vi "Begin.vi"(11 "Image Size":T1=enum."320x240") -> (0 "error out":errorcluster)   [LabVIEW 2011]
doc: "Called before other user functions, this VI is expected to open initial I/O refnums, load in file data, and do all program initialization. Notice that the <B>error out</B> terminal is simply used for data flow. Wiring it to other structures or subVIs ensures that this VI runs first."
uses:
  <vilib>/Rock Robotics/WPI/Camera/WPI_CameraImageSize.ctl
  <vilib>/Rock Robotics/SystemInterfaces/DIO/FPGA_DIOPWMChannel.ctl
  <vilib>/Rock Robotics/WPI/Joystick/WPI_JoystickDeviceEnum.ctl
  <vilib>/Rock Robotics/SystemInterfaces/DIO/FPGA_DIOChannel.ctl
  <vilib>/Rock Robotics/SystemInterfaces/DIO/FPGA_DIORelayChannel.ctl
  <vilib>/Rock Robotics/WPI/Solenoid/WPI_SolenoidChannel.ctl
  <vilib>/Rock Robotics/SystemInterfaces/Typedef/FPGA_TypedefAnalogModuleForGyro.ctl
  <vilib>/Rock Robotics/SystemInterfaces/AI/FPGA_AIGyroChannel.ctl
  <vilib>/Rock Robotics/SystemInterfaces/Typedef/FPGA_TypedefSolenoidModule.ctl
  <vilib>/Rock Robotics/SystemInterfaces/Typedef/FPGA_TypedefDigitalModule.ctl
  <vilib>/Rock Robotics/WPI/CAN/Jaguar/SubVIs/WPI_CANJaguar_ControlMode.ctl
  <vilib>/Rock Robotics/SystemInterfaces/Typedef/FPGA_TypedefAnalogModule.ctl
  <vilib>/Rock Robotics/SystemInterfaces/AI/FPGA_AIChannel.ctl
  <vilib>/Rock Robotics/WPI/Camera/WPI_CameraWhite Balance Values.ctl
  <vilib>/Rock Robotics/WPI/Camera/WPI_CameraExposure Values.ctl
  <vilib>/Rock Robotics/WPI/Encoder/WPI_EncoderType.ctl
  <vilib>/Rock Robotics/WPI/Camera/WPI_CameraFrameRate.ctl
  <vilib>/Rock Robotics/WPI/CAN/Jaguar/SubVIs/WPI_CANJaguar_BrakeCoastMode.ctl
  <vilib>/Rock Robotics/WPI/CAN/Jaguar/SubVIs/WPI_CANJaguar_LimitMode.ctl
  <vilib>/Rock Robotics/WPI/CAN/Jaguar/SubVIs/WPI_CANJaguar_PositionReference.ctl
  <vilib>/Rock Robotics/WPI/CAN/Jaguar/SubVIs/WPI_CANJaguar_StatusSelect.ctl
  <vilib>/Rock Robotics/WPI/CAN/Jaguar/SubVIs/WPI_CANJaguar_StatusChannelSelect.ctl
  <vilib>/Rock Robotics/WPI/RobotDrive/WPI_RobotDriveOpen4MotorWithVictor.vi
  <vilib>/Rock Robotics/WPI/Solenoid/WPI_SolenoidOpenSingle.vi
  <vilib>/Rock Robotics/WPI/MotorControl/WPI_MotorControlOpen Victor.vi
  <vilib>/Rock Robotics/WPI/RobotDrive/WPI_RobotDriveOpen2MotorWithExistingMotors.vi
  <vilib>/Rock Robotics/WPI/Counter/WPI_CounterDigitalInputToDigitalSource.vi
  Robot Global Data.vi
  <vilib>/Rock Robotics/WPI/MotorControl/WPI_MotorControlOpenCANJaguar.vi
  <vilib>/Rock Robotics/WPI/Compressor/WPI_CompressorGetSetRefNum.vi
panel:
  out "error out 2":errorcluster
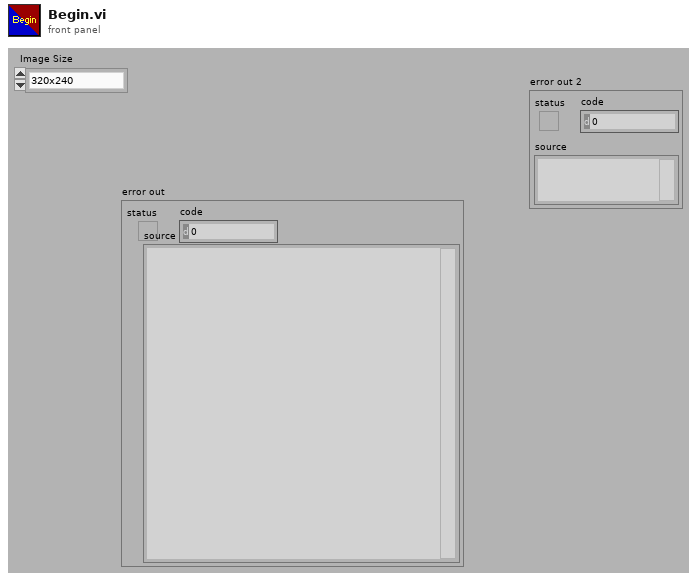
[diagram p1: front panel]
types:
  T1 = typedef "WPI_CameraImageSize.ctl" = enum16{"640x480", "320x240", "160x120"}
  T2 = typedef "WPI_CameraFrameRate.ctl" = u32
  T3 = typedef "FPGA_DIOChannel.ctl" = enum8{"DIO 1", "DIO 2", "DIO 3", "DIO 4", "DIO 5", "DIO 6", "DIO 7", "DIO 8", "DIO 9", "DIO 10", "DIO 11", "DIO 12", "DIO 13", "DIO 14", "Invalid"}
  T4 = typedef "FPGA_TypedefDigitalModule.ctl" = enum16{"Digital Module 1", "Digital Module 2"}
  T5 = typedef "WPI_EncoderType.ctl" = enum16{"1x", "2x", "4x"}
  T6 = typedef "WPI_CameraExposure Values.ctl" = enum16{"Auto", "Flicker-free 50 Hz", "Flicker-free 60 Hz", "Hold current"}
  T7 = typedef "WPI_CameraWhite Balance Values.ctl" = enum16{"Auto", "Fixed indoor", "Fixed outdoor 1", "Fixed outdoor 2", "Fixed fluorescent 1", "Fixed fluorescent 2", "Hold current"}
  T8 = typedef "WPI_SolenoidChannel.ctl" = enum8{"Solenoid 1", "Solenoid 2", "Solenoid 3", "Solenoid 4", "Solenoid 5", "Solenoid 6", "Solenoid 7", "Solenoid 8", "Invalid"}
  T9 = typedef "FPGA_TypedefSolenoidModule.ctl" = enum16{"Solenoid Module 1", "Solenoid Module 2"}
  T10 = typedef "FPGA_AIChannel.ctl" = enum8{"AI 1", "AI 2", "AI 3", "AI 4", "AI 5", "AI 6", "AI 7", "AI 8", "Invalid"}
  T11 = typedef "FPGA_TypedefAnalogModule.ctl" = enum16{"Analog Module 1", "Analog Module 2"}
  T12 = typedef "WPI_CANJaguar_ControlMode.ctl" = enum8{"Percent VBus", "Current", "Speed", "Position", "Voltage"}
  T13 = typedef "FPGA_DIOPWMChannel.ctl" = enum8{"PWM 1", "PWM 2", "PWM 3", "PWM 4", "PWM 5", "PWM 6", "PWM 7", "PWM 8", "PWM 9", "PWM 10", "Invalid"}
  T14 = typedef "FPGA_AIGyroChannel.ctl" = enum8{"AI 1", "AI 2", "Invalid"}
  T15 = typedef "FPGA_TypedefAnalogModuleForGyro.ctl" = enum16{"Analog Module 1"}
  T16 = typedef "WPI_JoystickDeviceEnum.ctl" = enum16{"USB 1", "USB 2", "USB 3", "USB 4", "Kinect 1", "Kinect 2"}
  T17 = typedef "FPGA_DIORelayChannel.ctl" = enum8{"Relay 1", "Relay 2", "Relay 3", "Relay 4", "Relay 5", "Relay 6", "Relay 7", "Relay 8", "Invalid"}
  T18 = typedef "WPI_AnalogChannelDevRef.ctl" = cluster{"DevStatus":errorcluster, "Analog Module":T11, "Analog Channel":T10}
  T19 = typedef "WPI_DigitalInputDevRef.ctl" = cluster{"DevStatus":errorcluster, "DIO Channel":T3, "Digital Module":T4}
  T20 = typedef "WPI_GyroDevRef.ctl" = cluster{"DevStatus":errorcluster, "Analog Module":T11, "Analog Channel":T10, "Offset":dbl, "Gain (VoltsPerDegree/Second)":dbl}
  T21 = typedef "FPGA_CounterEncoderSourceConvertionLVSourceType.ctl" = cluster{"DevStatus":errorcluster, "AnalogTriggerMode?":bool, "DigitalMode":cluster{"Digital Module":T4, "DIO Channel":T22}, "AnalogTriggerMode":cluster{"AnalogTriggerIndex":T23, "OutputType":T24}}
  T22 = typedef "FPGA_DIODigitalSourceChannel.ctl" = enum8{"DIO 1", "DIO 2", "DIO 3", "DIO 4", "DIO 5", "DIO 6", "DIO 7", "DIO 8", "DIO 9", "DIO 10", "DIO 11", "DIO 12", "DIO 13", "DIO 14", "Disabled"}
  T23 = typedef "FPGA_AnalogTriggerIndex.ctl" = enum8{"Trig 0", "Trig 1", "Trig 2", "Trig 3", "Trig 4", "Trig 5", "Trig 6", "Trig 7", "Invalid"}
  T24 = typedef "FPGA_AnalogTriggerOutType.ctl" = enum16{"InWindow", "TriggerState", "Rising", "Falling"}
  T25 = typedef "WPI_EncoderDevRef.ctl" = cluster{"DevStatus":errorcluster, "EncoderIndex":T26, "CounterIndex":T27, "DistancePerCount":dbl, "Decoding Type":T5}
  T26 = typedef "FPGA_EncoderIdx.ctl" = enum8{"Enc 0", "Enc 1", "Enc 2", "Enc 3", "Invalid"}
  T27 = typedef "FPGA_CounterCtrSystemIndex.ctl" = enum8{"Ctr 0", "Ctr 1", "Ctr 2", "Ctr 3", "Ctr 4", "Ctr 5", "Ctr 6", "Ctr 7", "Invalid"}
  T28 = typedef "WPI_CameraDevRef.ctl" = cluster{"Camera Address":string, "CameraStatus":errorcluster, "Acquire Image Notifier":refnum<notifier>}
  T29 = typedef "WPI_CompressorDevRef.ctl" = cluster{"DevStatus":errorcluster, "DigitalInputDevRef":T19, "RelayDevRef":T30}
  T30 = typedef "WPI_RelayDevRef.ctl" = cluster{"DevStatus":errorcluster, "Relay Channel":T17, "Digital Module":T4, "Relay Direction":T31}
  T31 = typedef "WPI_RelayDirection.ctl" = enum16{"Both directions", "Forward only", "Reverse only"}
  T32 = typedef "WPI_MotorControlDeviceRef.ctl" = cluster{"DeviceStatus":errorcluster, "Type":enum16{"PWM", "CAN"}, "PWM":cluster{"Digital Module":T4, "PWM Channel":T13, "DeadBand":T33}, "CAN":cluster{"Device Number":u8, "Control Mode":T12, "Semaphore":T34, "Max Vout":dbl}, "Invert":bool, "TransformRef":T35, "InvTransformRef":T35}
  T33 = typedef "WPI_PWMDeadband.ctl" = cluster{"Name":string, "maxPositivePwm":i32, "minPositivePwm":i32, "centerPwm":i32, "maxNegativePwm":i32, "minNegativePwm":i32, "angularRange":u16}
  T34 = typedef "Semaphore RefNum" = refnum<k1>
  T35 = typedef "WPI_PWMTransform_ConPane.ctl" = refnum<vi>
  T36 = typedef "WPI_DigitalOutputDevRef.ctl" = cluster{"Digital Module":T4, "DIO Channel":T3, "DevStatus":errorcluster}
  T37 = typedef "WPI_SolenoidDevRef.ctl" = cluster{"DevStatus":errorcluster, "Solenoid Module":T9, "Forward Solenoid Channel":T8, "Reverse Solenoid Channel":T8}
  T38 = typedef "WPI_JoystickDevRef.ctl" = cluster{"Device":T16}
  T39 = typedef "WPI_RobotDriveDevRef.ctl" = cluster{"DevStatus":errorcluster, "Motors[]":T32[], "Square Inputs":bool, "Max Output":dbl, "Isochronous":bool}
  T40 = typedef "WPI_CANJaguar_BrakeCoastMode.ctl" = enum8{"Jumper", "Brake", "Coast"}
  T41 = typedef "WPI_CANJaguar_LimitMode.ctl" = enum16{"Switch Inputs Only", "Soft Position Limits"}
  T42 = typedef "WPI_CANJaguar_StatusChannelSelect.ctl" = enum16{"Periodic Status Channel 1", "Periodic Status Channel 2", "Periodic Status Channel 3", "Periodic Status Channel 4", "On Demand Status"}
  T43 = typedef "WPI_CANJaguar_PositionReference.ctl" = u8
  T44 = typedef "WPI_CANJaguar_StatusSelect.ctl" = enum16{"Output Percent VBus", "Output Voltage", "Bus Voltage", "Current", "Temperature", "Position", "Speed", "Limit Switches", "Faults", "Fault Counters", "Power Cycle"}
  T45 = typedef "InitCounts.ctl" = cluster{"Top Shooter":i8, "Bottom Shooter ":i8, "Turret":i8, "Stage 2":i8}
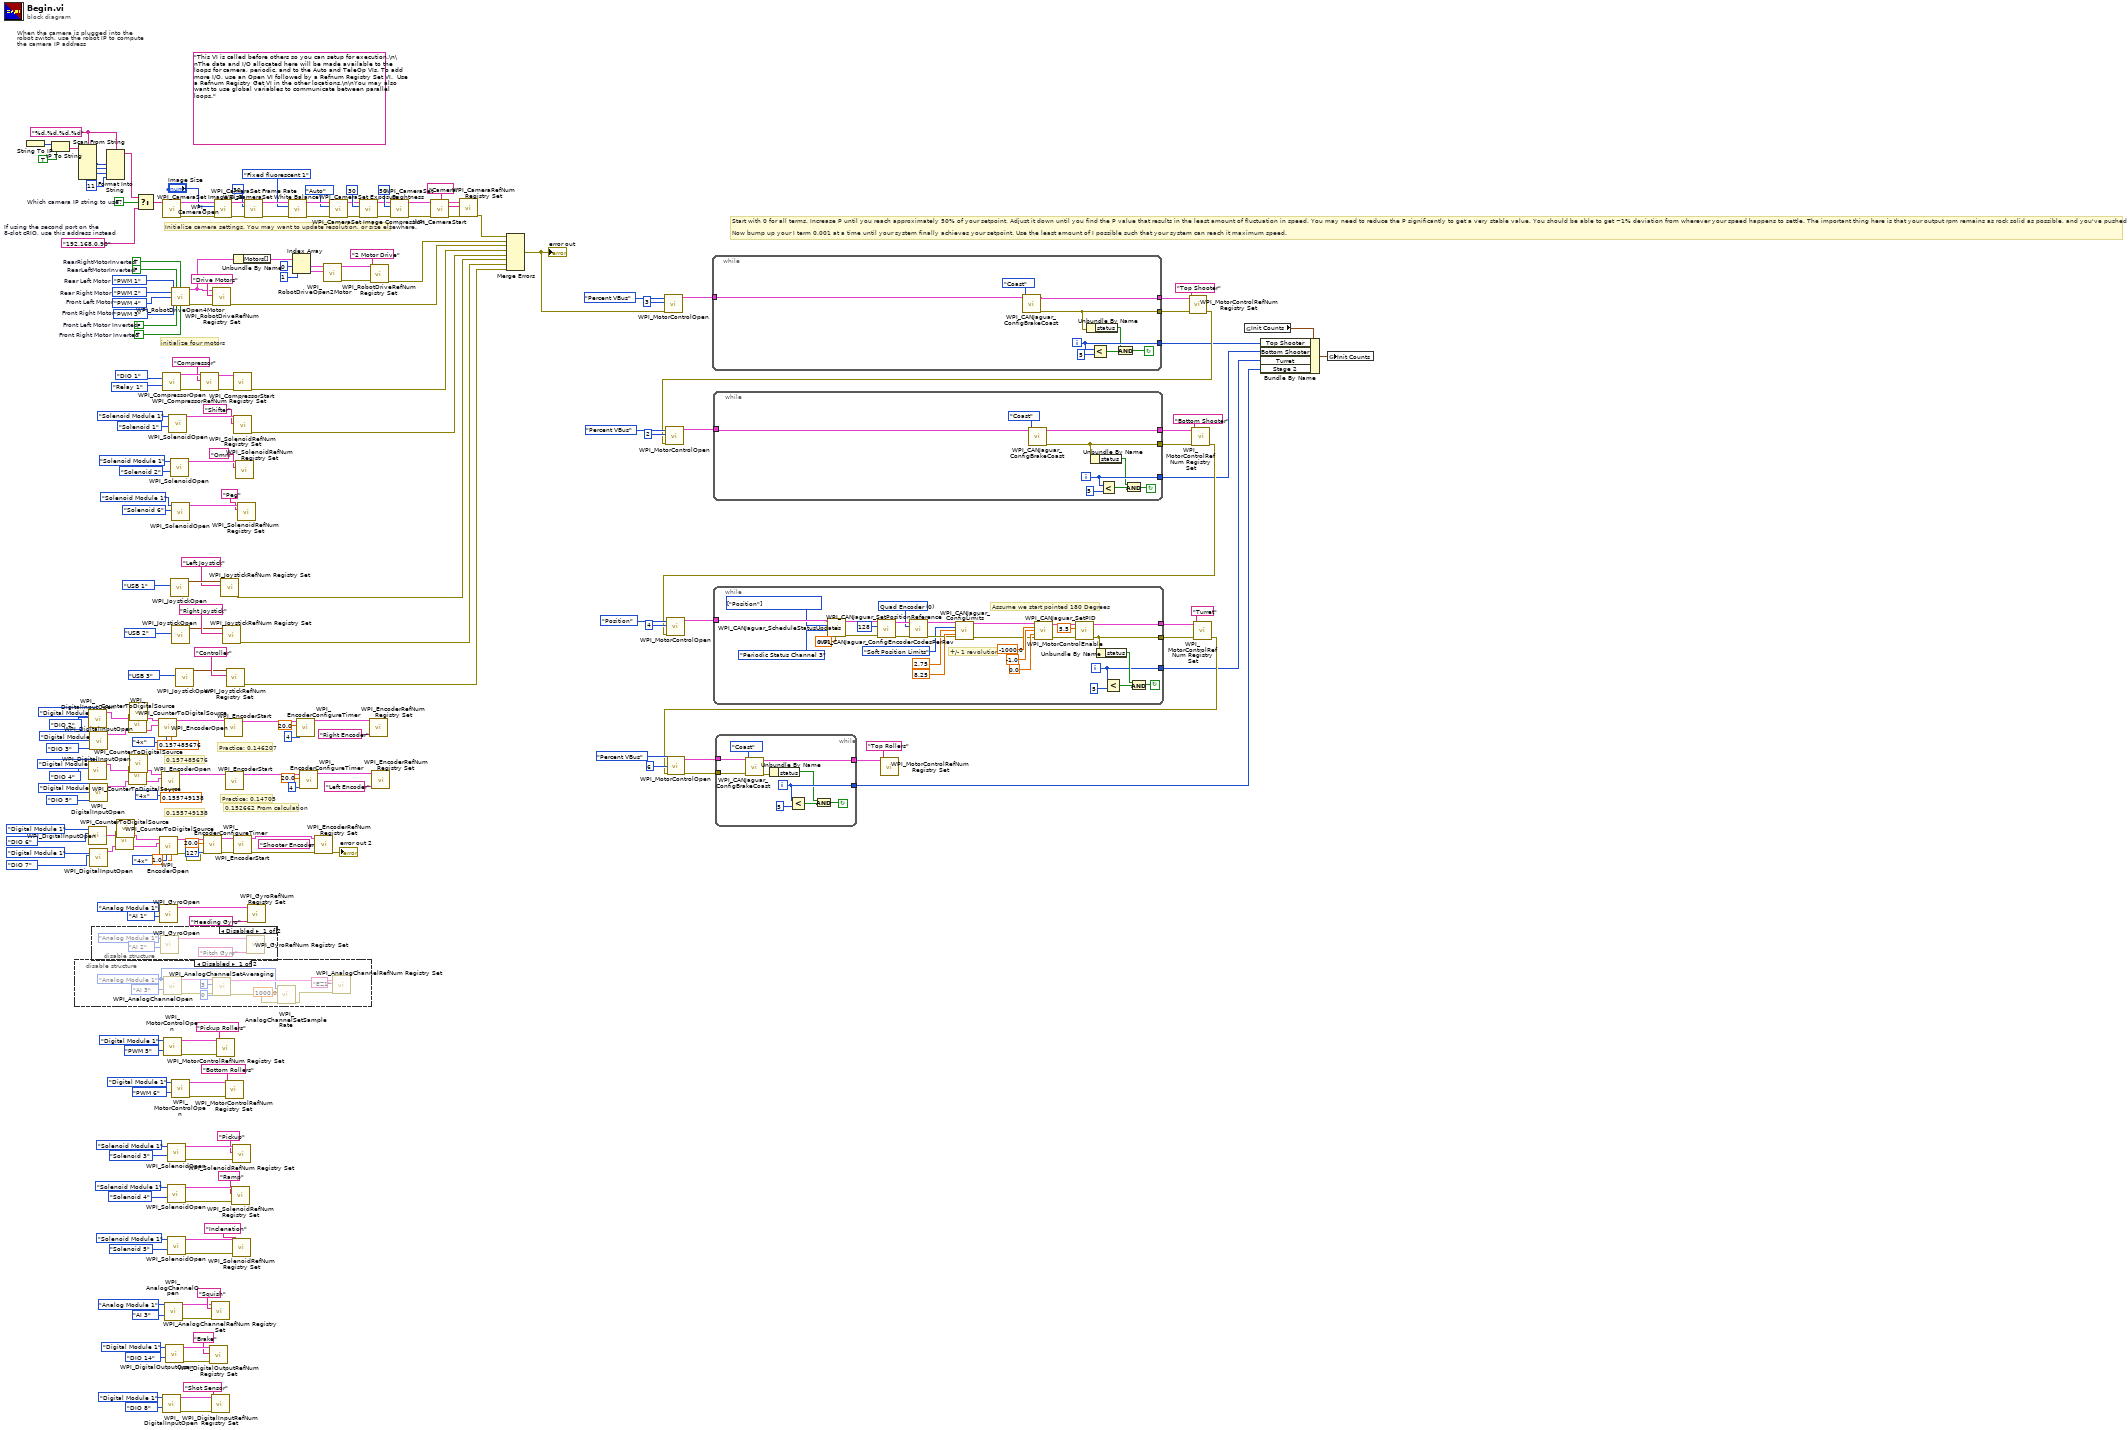
[diagram p0: block diagram]
diagram:
  w60 = TRUE  # Which camera IP string to use?
  w63 = "%d.%d.%d.%d" ("format string")
  (unwired) "This VI is called before others so you can setup for execution.\n\nThe data and I/O allocated here will be made available to the loops for camera, periodic, and to the Auto and TeleOp VIs. To add more I/O, use an Open VI followed by a Refnum Registry Set VI.  Use a Refnum Registry Get VI in the other locations.\n\nYou may also want to use global variables to communicate between parallel loops."
  w75 = "192.168.0.90"  # If using the second port on the 8-slot cRIO, use this address instead
  w205 = TRUE  # Front Right Motor Inverted
  w206 = FALSE  # Front Left Motor Inverted
  w207 = FPGA_DIOPWMChannel."PWM 3"  # Front Right Motor
  w208 = FPGA_DIOPWMChannel."PWM 4"  # Front Left Motor
  w213 = FPGA_DIOPWMChannel."PWM 2"  # Rear Right Motor
  w214 = FPGA_DIOPWMChannel."PWM 1"  # Rear Left Motor
  w219 = FALSE  # RearLeftMotorInverted
  w220 = TRUE  # RearRightMotorInverted
  # "Practice: 0.14705"
  # "Practice: 0.146207"
  # "0.155749138"
  # "0.157485676"
  # "0.152662 From calculation"
  # "Initialize camera settings. You may want to update resolution, or size elsewhere."
  # "When the camera is plugged into the\nrobot switch, use the robot IP to compute\nthe camera IP address"
  # "Start with 0 for all terms. Increase P until you reach approximately 50% of your setpoint. Adjust it down until you find the P value that results in the least amount of fluctuation in speed. You may need to reduce the P significantly to get a very stable value. You should be able to get ~1% deviation from wherever your speed happens to settle. The important thing here is that your output rpm remains as rock solid as possible, and you've pushed it as close to 50% of your setpoint as you can get it.\n\nNow bump up your I term 0.001 at a time until your system finally achieves your setpoint. Use the least amount of I possible such that your system can reach it maximum speed."
  # "initialize four motors"
  n1 = String To IP() -> (0:w70:u32)  [unwired: 1 in]
  n2 = IP To String(1:TRUE ("dot notation? (F)"), 2:w70) -> (0:w68:string)
  n3 = disable-structure shown="Disabled" {
    frame Disabled {
      w221 = FPGA_TypedefAnalogModule."Analog Module 1" ("Analog Module (Module 1)")
      n4 = call <vilib>:"WPI_AnalogChannelOpen.vi"("Analog Channel"=FPGA_AIChannel."AI 3", "Analog Module (Module 1)"=w221) -> ("error out"=w228:errorcluster, "AIDeviceRef"=w229:T18)  [unwired: 8 in]
      n5 = call <vilib>:"WPI_AnalogChannelSetAveraging.vi"("error in (no error)"=w228, "OversampleBits"=u8 0, "AverageBits"=u8 3, "AIDeviceRef"=w229) -> ("error out"=w227:errorcluster, "AIDeviceRef"=w226:T18)  [unwired: 6 out]
      n6 = call <vilib>:"WPI_AnalogChannelSetSampleRate.vi"("error in (no error)"=w227, "Samples Per Second"=1000.0, "Analog Module (Module 1)"=w221) -> ("error out"=w225:errorcluster)  [unwired: 1 in, 7 out]
      n7 = call <vilib>:"WPI_AnalogChannelRefNum Registry Set.vi"("error in (no error)"=w225, "refnum name"="EZ1", "AIDeviceRef"=w226) -> ()  [unwired: 7 in, 2 out]
    }
    frame Enabled {
    }
  }
  n8 = Scan From String(format string=w63, input string=w68) -> (output 1=w67:i32, output 2=w66:i32, output 3=w65:i32)  [unwired: 7 in, 3 out]
  n9 = call <vilib>:"WPI_DigitalInputOpen.vi"("DIO Channel"=FPGA_DIOChannel."DIO 4", "Digital Module (Module 1)"=FPGA_TypedefDigitalModule."Digital Module 1" ("DIO Module (Slot 4)")) -> ("DigitalInputDevRef"=w9:T19)  [unwired: 1 in, 8 out]
  n10 = call <vilib>:"WPI_DigitalInputOpen.vi"("DIO Channel"=FPGA_DIOChannel."DIO 6", "Digital Module (Module 1)"=FPGA_TypedefDigitalModule."Digital Module 1" ("DIO Module (Slot 4)")) -> ("DigitalInputDevRef"=w86:T19)  [unwired: 1 in, 8 out]
  n11 = call <vilib>:"WPI_DigitalInputOpen.vi"("DIO Channel"=FPGA_DIOChannel."DIO 2", "Digital Module (Module 1)"=FPGA_TypedefDigitalModule."Digital Module 1" ("DIO Module (Slot 4)")) -> ("DigitalInputDevRef"=w18:T19)  [unwired: 1 in, 8 out]
  n12 = call <vilib>:"WPI_DigitalInputOpen.vi"("DIO Channel"=FPGA_DIOChannel."DIO 5", "Digital Module (Module 1)"=FPGA_TypedefDigitalModule."Digital Module 1" ("DIO Module (Slot 4)")) -> ("DigitalInputDevRef"=w6:T19)  [unwired: 1 in, 8 out]
  n13 = call <vilib>:"WPI_DigitalInputOpen.vi"("DIO Channel"=FPGA_DIOChannel."DIO 7", "Digital Module (Module 1)"=FPGA_TypedefDigitalModule."Digital Module 1" ("DIO Module (Slot 4)")) -> ("DigitalInputDevRef"=w89:T19)  [unwired: 1 in, 8 out]
  n14 = call <vilib>:"WPI_DigitalInputOpen.vi"("DIO Channel"=FPGA_DIOChannel."DIO 3", "Digital Module (Module 1)"=FPGA_TypedefDigitalModule."Digital Module 1" ("DIO Module (Slot 4)")) -> ("DigitalInputDevRef"=w13:T19)  [unwired: 1 in, 8 out]
  n15 = disable-structure shown="Disabled" {
    frame Disabled {
      n16 = call <vilib>:"WPI_GyroOpen.vi"("Analog Channel"=FPGA_AIGyroChannel."AI 2", "Analog Module (Module 1)"=FPGA_TypedefAnalogModuleForGyro."Analog Module 1" ("Analog Module (Slot 1)")) -> ("GyroDevRef"=w235:T20)  [unwired: 4 in, 5 out]
      n17 = call <vilib>:"WPI_GyroRefNum Registry Set.vi"("refnum name"="Pitch Gyro", "GyroDevRef"=w235) -> ()  [unwired: 1 in, 9 out]
    }
    frame Enabled {
    }
  }
  n18 = Format Into String(format string=w63, w67, w66, w65, 11 ("Compression")) -> (resulting string=w61:string)  [unwired: 2 in, 1 out]
  n19 = call-poly <vilib>:"WPI_CounterToDigitalSource.vi"("DigitalInputDevRef"=w89) -> ("Digital Source"=w91:T21)  [unwired: 6 out]
  n20 = call-poly <vilib>:"WPI_CounterToDigitalSource.vi"("DigitalInputDevRef"=w86) -> ("Digital Source"=w90:T21)  [unwired: 6 out]
  n21 = call-poly <vilib>:"WPI_CounterToDigitalSource.vi"("DigitalInputDevRef"=w6) -> ("Digital Source"=w4:T21)  [unwired: 6 out]
  n22 = call-poly <vilib>:"WPI_CounterToDigitalSource.vi"("DigitalInputDevRef"=w13) -> ("Digital Source"=w14:T21)  [unwired: 6 out]
  n23 = call-poly <vilib>:"WPI_CounterToDigitalSource.vi"("DigitalInputDevRef"=w9) -> ("Digital Source"=w5:T21)  [unwired: 6 out]
  n24 = call-poly <vilib>:"WPI_CounterToDigitalSource.vi"("DigitalInputDevRef"=w18) -> ("Digital Source"=w19:T21)  [unwired: 6 out]
  n25 = Select(t=w61, s=w60, f=w75) -> (s? t:f=w62:string)
  n26 = call <vilib>:"WPI_EncoderOpen.vi"("DistancePerCount"=0.157485676, "Decoding Type"=WPI_EncoderType."4x", "BSource"=w14, "ASource"=w19) -> ("EncoderDevRef"=w33:T25)  [unwired: 4 in, 3 out]
  n27 = call <vilib>:"WPI_EncoderOpen.vi"("DistancePerCount"=1.0, "Decoding Type"=WPI_EncoderType."4x", "BSource"=w91, "ASource"=w90) -> ("error out"=w40:errorcluster, "EncoderDevRef"=w39:T25)  [unwired: 4 in, 2 out]
  n28 = call <vilib>:"WPI_GyroOpen.vi"("Analog Channel"=FPGA_AIGyroChannel."AI 1", "Analog Module (Module 1)"=FPGA_TypedefAnalogModuleForGyro."Analog Module 1" ("Analog Module (Slot 1)")) -> ("GyroDevRef"=w181:T20)  [unwired: 4 in, 5 out]
  n29 = call <vilib>:"WPI_EncoderOpen.vi"("DistancePerCount"=0.155749138, "Decoding Type"=WPI_EncoderType."4x", "BSource"=w4, "ASource"=w5) -> ("EncoderDevRef"=w30:T25)  [unwired: 4 in, 3 out]
  n30 = call <vilib>:"WPI_DigitalInputOpen.vi"("DIO Channel"=FPGA_DIOChannel."DIO 8", "Digital Module (Module 1)"=FPGA_TypedefDigitalModule."Digital Module 1") -> ("error out"=w77:errorcluster, "DigitalInputDevRef"=w78:T19)  [unwired: 8 in]
  n31 = call <vilib>:"WPI_CameraOpen.vi"("Camera Address"=w62) -> ("error out"=w72:errorcluster, "CameraDevRef"=w73:T28)  [unwired: 1 in, 8 out]
  n32 = call <vilib>:"WPI_CompressorOpen.vi"("Pressure Switch DIO Channel"=FPGA_DIOChannel."DIO 1", "Relay Channel"=FPGA_DIORelayChannel."Relay 1") -> ("CompressorDevRef"=w204:T29, "error out"=w203:errorcluster)  [unwired: 12 in]
  n33 = call-poly <vilib>:"WPI_MotorControlOpen.vi"("PWM Channel"=FPGA_DIOPWMChannel."PWM 5", "Digital Module (Module 1)"=FPGA_TypedefDigitalModule."Digital Module 1") -> ("error out"=w171:errorcluster, "MotorControlDeviceRef"=w172:T32)  [unwired: 8 in]
  n34 = call <vilib>:"WPI_AnalogChannelOpen.vi"("Analog Channel"=FPGA_AIChannel."AI 3", "Analog Module (Module 1)"=FPGA_TypedefAnalogModule."Analog Module 1") -> ("error out"=w115:errorcluster, "AIDeviceRef"=w116:T18)  [unwired: 8 in]
  n35 = call <vilib>:"WPI_DigitalOutputOpen.vi"("DIO Channel"=FPGA_DIOChannel."DIO 14", "Digital Module (Module 1)"=FPGA_TypedefDigitalModule."Digital Module 1") -> ("error out"=w113:errorcluster, "DigitalOutputDevRef"=w114:T36)  [unwired: 8 in]
  n36 = call-poly <vilib>:"WPI_SolenoidOpen.vi"("Solenoid Channel"=WPI_SolenoidChannel."Solenoid 4", "Solenoid Module (Module 1)"=FPGA_TypedefSolenoidModule."Solenoid Module 1" ("Solenoid Module")) -> ("error out"=w157:errorcluster, "SolenoidDevRef"=w161:T37)  [unwired: 1 in, 7 out]
  n37 = call-poly <vilib>:"WPI_SolenoidOpen.vi"("Solenoid Channel"=WPI_SolenoidChannel."Solenoid 3", "Solenoid Module (Module 1)"=FPGA_TypedefSolenoidModule."Solenoid Module 1" ("Solenoid Module")) -> ("error out"=w162:errorcluster, "SolenoidDevRef"=w180:T37)  [unwired: 1 in, 7 out]
  n38 = call-poly <vilib>:"WPI_SolenoidOpen.vi"("Solenoid Channel"=WPI_SolenoidChannel."Solenoid 5", "Solenoid Module (Module 1)"=FPGA_TypedefSolenoidModule."Solenoid Module 1" ("Solenoid Module")) -> ("error out"=w151:errorcluster, "SolenoidDevRef"=w147:T37)  [unwired: 1 in, 7 out]
  n39 = call-poly <vilib>:"WPI_SolenoidOpen.vi"("Solenoid Channel"=WPI_SolenoidChannel."Solenoid 1", "Solenoid Module (Module 1)"=FPGA_TypedefSolenoidModule."Solenoid Module 1" ("Solenoid Module")) -> ("SolenoidDevRef"=w197:T37)  [unwired: 1 in, 8 out]
  n40 = call-poly <vilib>:"WPI_SolenoidOpen.vi"("Solenoid Channel"=WPI_SolenoidChannel."Solenoid 2", "Solenoid Module (Module 1)"=FPGA_TypedefSolenoidModule."Solenoid Module 1" ("Solenoid Module")) -> ("SolenoidDevRef"=w176:T37)  [unwired: 1 in, 8 out]
  n41 = call <vilib>:"WPI_JoystickOpen.vi"("JoystickDevice"=WPI_JoystickDeviceEnum."USB 1") -> ("JoystickDevRef"=w217:T38)  [unwired: 10 out]
  n42 = call-poly <vilib>:"WPI_RobotDriveOpen4Motor.vi"("Rear Left Motor"=w214, "Rear Left Motor Inverted"=w219, "Rear Right Motor Inverted"=w220, "Rear Right Motor"=w213, "Front Left Motor"=w208, "Front Right Motor"=w207, "Front Left Motor Inverted"=w206, "Front Right Motor Inverted"=w205) -> ("RobotDriveDevRef"=w146:T39, "error out"=w215:errorcluster)  [unwired: 6 in]
  n43 = call-poly <vilib>:"WPI_SolenoidOpen.vi"("Solenoid Channel"=WPI_SolenoidChannel."Solenoid 6", "Solenoid Module (Module 1)"=FPGA_TypedefSolenoidModule."Solenoid Module 1") -> ("SolenoidDevRef"=w94:T37)  [unwired: 8 in, 1 out]
  n44 = call <vilib>:"WPI_JoystickOpen.vi"("JoystickDevice"=WPI_JoystickDeviceEnum."USB 2") -> ("JoystickDevRef"=w209:T38)  [unwired: 10 out]
  n45 = call-poly <vilib>:"WPI_MotorControlOpen.vi"("PWM Channel"=FPGA_DIOPWMChannel."PWM 6", "Digital Module (Module 1)"=FPGA_TypedefDigitalModule."Digital Module 1") -> ("error out"=w166:errorcluster, "MotorControlDeviceRef"=w167:T32)  [unwired: 8 in]
  n46 = call <vilib>:"WPI_JoystickOpen.vi"("JoystickDevice"=WPI_JoystickDeviceEnum."USB 3") -> ("JoystickDevRef"=w191:T38)  [unwired: 10 out]
  n47 = call <vilib>:"WPI_CompressorRefNum Registry Set.vi"("error in (no error)"=w203, "refnum name"="Compressor", "CompressorDevRef"=w204) -> ("error out"=w200:errorcluster, "CompressorDevRef"=w201:T29)  [unwired: 7 in]
  n48 = call <vilib>:"WPI_EncoderConfigureTimer.vi"("error in (no error)"=w40, "Number Samples to Average"=u8 127, "Minimum Rate"=20.0, "EncoderDevRef"=w39) -> ("error out"=w38:errorcluster, "EncoderDevRef"=w37:T25)  [unwired: 6 out]
  n49 = call <vilib>:"WPI_DigitalOutputRefNum Registry Set.vi"("error in (no error)"=w113, "refnum name"="Brake", "DigitalOutputDevRef"=w114) -> ()  [unwired: 7 in, 2 out]
  n50 = call <vilib>:"WPI_AnalogChannelRefNum Registry Set.vi"("error in (no error)"=w115, "refnum name"="Squish", "AIDeviceRef"=w116) -> ()  [unwired: 7 in, 2 out]
  n51 = call <vilib>:"WPI_DigitalInputRefNum Registry Set.vi"("error in (no error)"=w77, "refnum name"="Shot Sensor", "DigitalInputDevRef"=w78) -> ()  [unwired: 7 in, 2 out]
  n52 = call <vilib>:"WPI_RobotDriveRefNum Registry Set.vi"("error in (no error)"=w215, "refnum name"="Drive Motors", "RobotDriveDevRef"=w146) -> ("error out"=w190:errorcluster)  [unwired: 8 out]
  n53 = call <vilib>:"WPI_CameraSet Image Size.vi"("error in (no error)"=w72, "Image Size"="Image Size", "CameraDevRef"=w73) -> ("error out"=w52:errorcluster, "CameraDevRef Out"=w53:T28)  [unwired: 7 out]
  n54 = call <vilib>:"WPI_MotorControlRefNum Registry Set.vi"("error in (no error)"=w171, "refnum name"="Pickup Rollers", "MotorControlDevRef"=w172) -> ()  [unwired: 7 in, 2 out]
  n55 = call <vilib>:"WPI_JoystickRefNum Registry Set.vi"("refnum name"="Left Joystick", "JoystickDevRef"=w217) -> ("error out"=w187:errorcluster)  [unwired: 1 in, 8 out]
  n56 = call <vilib>:"WPI_JoystickRefNum Registry Set.vi"("refnum name"="Right Joystick", "JoystickDevRef"=w209) -> ("error out"=w186:errorcluster)  [unwired: 1 in, 8 out]
  n57 = call <vilib>:"WPI_EncoderStart.vi"("EncoderDevRef"=w33) -> ("EncoderDevRef"=w32:T25)  [unwired: 1 in, 9 out]
  n58 = call <vilib>:"WPI_MotorControlRefNum Registry Set.vi"("error in (no error)"=w166, "refnum name"="Bottom Rollers", "MotorControlDevRef"=w167) -> ()  [unwired: 7 in, 2 out]
  n59 = call <vilib>:"WPI_EncoderStart.vi"("EncoderDevRef"=w30) -> ("EncoderDevRef"=w29:T25)  [unwired: 1 in, 9 out]
  n60 = call <vilib>:"WPI_JoystickRefNum Registry Set.vi"("refnum name"="Controller", "JoystickDevRef"=w191) -> ("error out"=w185:errorcluster)  [unwired: 1 in, 8 out]
  n61 = call <vilib>:"WPI_SolenoidRefNum Registry Set.vi"("error in (no error)"=w157, "refnum name"="Ramp", "SolenoidDevRef"=w161) -> ()  [unwired: 9 out]
  n62 = call <vilib>:"WPI_SolenoidRefNum Registry Set.vi"("error in (no error)"=w162, "refnum name"="Pickup", "SolenoidDevRef"=w180) -> ()  [unwired: 9 out]
  n63 = call <vilib>:"WPI_SolenoidRefNum Registry Set.vi"("error in (no error)"=w151, "refnum name"="Inclenation", "SolenoidDevRef"=w147) -> ()  [unwired: 9 out]
  n64 = call <vilib>:"WPI_CompressorStart.vi"("error in (no error)"=w200, "CompressorDevRef"=w201) -> ("error out"=w189:errorcluster)  [unwired: 8 in, 1 out]
  n65 = call <vilib>:"WPI_EncoderStart.vi"("error in (no error)"=w38, "EncoderDevRef"=w37) -> ("error out"=w36:errorcluster, "EncoderDevRef"=w35:T25)  [unwired: 8 in]
  n66 = Unbundle By Name(w146) -> ("Motors[]"=w145:T32[])
  n67 = call <vilib>:"WPI_SolenoidRefNum Registry Set.vi"("refnum name"="Shifter", "SolenoidDevRef"=w197) -> ("error out"=w188:errorcluster)  [unwired: 1 in, 8 out]
  n68 = call <vilib>:"WPI_SolenoidRefNum Registry Set.vi"("refnum name"="Omni", "SolenoidDevRef"=w176) -> ()  [unwired: 1 in, 9 out]
  n69 = call <vilib>:"WPI_SolenoidRefNum Registry Set.vi"("refnum name"="Peg", "SolenoidDevRef"=w94) -> ()  [unwired: 8 in, 2 out]
  n70 = call <vilib>:"WPI_CameraSet Frame Rate.vi"("error in (no error)"=w52, "Frame Rate (fps)"=T2 30, "CameraDevRef"=w53) -> ("error out"=w51:errorcluster, "CameraDevRef Out"=w55:T28)  [unwired: 7 out]
  n71 = call <vilib>:"WPI_GyroRefNum Registry Set.vi"("refnum name"="Heading Gyro", "GyroDevRef"=w181) -> ()  [unwired: 1 in, 9 out]
  n72 = call <vilib>:"WPI_CameraSet White Balance.vi"("error in (no error)"=w51, "White Balance"=WPI_CameraWhite_Balance_Values."Fixed fluorescent 1", "CameraDevRef"=w55) -> ("error out"=w50:errorcluster, "CameraDevRef Out"=w54:T28)  [unwired: 7 out]
  n73 = Index Array(array=w145, index #1=0 ("index"), index #2=1 ("index")) -> (element #1=w142:T32, element #2=w141:T32)
  n74 = call <vilib>:"WPI_EncoderConfigureTimer.vi"("Number Samples to Average"=u8 4, "Minimum Rate"=20.0, "EncoderDevRef"=w32) -> ("EncoderDevRef"=w31:T25)  [unwired: 1 in, 7 out]
  n75 = call <vilib>:"WPI_EncoderConfigureTimer.vi"("Number Samples to Average"=u8 4, "Minimum Rate"=20.0, "EncoderDevRef"=w29) -> ("EncoderDevRef"=w28:T25)  [unwired: 1 in, 7 out]
  n76 = call <vilib>:"WPI_EncoderRefNum Registry Set.vi"("error in (no error)"=w36, "refnum name"="Shooter Encoder", "EncoderDevRef"=w35) -> ("error out"=→"error out 2":errorcluster)  [unwired: 8 out]
  n77 = call-poly <vilib>:"WPI_RobotDriveOpen2Motor.vi"("Right Motor Dev Ref"=w141, "Left Motor Dev Ref"=w142) -> ("error out"=w139:errorcluster, "RobotDriveDevRef"=w140:T39)  [unwired: 8 in]
  n78 = call <vilib>:"WPI_CameraSet Exposure.vi"("error in (no error)"=w50, "Exposure"=WPI_CameraExposure_Values."Auto", "CameraDevRef"=w54) -> ("error out"=w49:errorcluster, "CameraDevRef Out"=w57:T28)  [unwired: 7 out]
  n79 = call <vilib>:"WPI_CameraSet Image Compression.vi"("error in (no error)"=w49, "Compression"=30, "CameraDevRef"=w57) -> ("error out"=w48:errorcluster, "CameraDevRef Out"=w56:T28)  [unwired: 7 out]
  n80 = call <vilib>:"WPI_EncoderRefNum Registry Set.vi"("refnum name"="Right Encoder", "EncoderDevRef"=w31) -> ()  [unwired: 1 in, 9 out]
  n81 = call <vilib>:"WPI_RobotDriveRefNum Registry Set.vi"("error in (no error)"=w139, "refnum name"="2 Motor Drive", "RobotDriveDevRef"=w140) -> ("error out"=w136:errorcluster)  [unwired: 8 out]
  n82 = call <vilib>:"WPI_EncoderRefNum Registry Set.vi"("refnum name"="Left Encoder", "EncoderDevRef"=w28) -> ()  [unwired: 1 in, 9 out]
  n83 = call <vilib>:"WPI_CameraSet Brightness.vi"("error in (no error)"=w48, "Brightness"=50, "CameraDevRef"=w56) -> ("error out"=w44:errorcluster, "CameraDevRef Out"=w45:T28)  [unwired: 7 out]
  n84 = call <vilib>:"WPI_CameraStart.vi"("error in (no error)"=w44, "CameraDevRef"=w45) -> ("error out"=w42:errorcluster, "CameraDevRef Out"=w43:T28)  [unwired: 8 in]
  n85 = call <vilib>:"WPI_CameraRefNum Registry Set.vi"("error in (no error)"=w42, "refnum name"="Camera", "CameraDevRef"=w43) -> ("error out"=w137:errorcluster)  [unwired: 8 out]
  n86 = Merge Errors(w137, w136, w190, w189, w188, w187, w186, w185) -> (w97:errorcluster)
  "error out" <- w97
  n87 = call-poly <vilib>:"WPI_MotorControlOpen.vi"("error in (no error)"=w97, "Device Number"=u8 3, "Control Mode"=WPI_CANJaguar_ControlMode."Percent VBus") -> ("MotorControlDeviceRef"=w132:T32)  [unwired: 7 in, 1 out]
  n88 = while {
    tunnel: w132 -> [w236]
    tunnel: [w237] -> w131
    tunnel: [w238] -> w109
    tunnel: [w243] -> w101
    i -> [w243]
    stop <- w240 continue-if-true
    n89 = call <vilib>:"WPI_CANJaguar_ConfigBrakeCoast.vi"("Brake / Coast Mode"=WPI_CANJaguar_BrakeCoastMode."Coast", "CAN Jaguar Ref"=w236) -> ("error out"=w238:errorcluster, "CAN Jaguar Ref Out"=w237:T32)  [unwired: 8 in]
    n90 = Unbundle By Name(w238) -> ("status"=w239:bool)
    n91 = Less?(x=w243, y=5) -> (x < y?=w241:bool)
    n92 = And(x=w239, y=w241) -> (x .and. y?=w240:bool)
  }
  n93 = call <vilib>:"WPI_MotorControlRefNum Registry Set.vi"("error in (no error)"=w109, "refnum name"="Top Shooter", "MotorControlDevRef"=w131) -> ("error out"=w106:errorcluster)  [unwired: 7 in, 1 out]
  n94 = call-poly <vilib>:"WPI_MotorControlOpen.vi"("error in (no error)"=w106, "Device Number"=u8 2, "Control Mode"=WPI_CANJaguar_ControlMode."Percent VBus") -> ("MotorControlDeviceRef"=w127:T32)  [unwired: 7 in, 1 out]
  n95 = while {
    tunnel: w127 -> [w247]
    tunnel: [w245] -> w126
    tunnel: [w246] -> w108
    tunnel: [w250] -> w100
    i -> [w250]
    stop <- w249 continue-if-true
    n96 = call <vilib>:"WPI_CANJaguar_ConfigBrakeCoast.vi"("Brake / Coast Mode"=WPI_CANJaguar_BrakeCoastMode."Coast", "CAN Jaguar Ref"=w247) -> ("error out"=w246:errorcluster, "CAN Jaguar Ref Out"=w245:T32)  [unwired: 8 in]
    n97 = Unbundle By Name(w246) -> ("status"=w248:bool)
    n98 = Less?(x=w250, y=5) -> (x < y?=w251:bool)
    n99 = And(x=w248, y=w251) -> (x .and. y?=w249:bool)
  }
  n100 = call <vilib>:"WPI_MotorControlRefNum Registry Set.vi"("error in (no error)"=w108, "refnum name"="Bottom Shooter", "MotorControlDevRef"=w126) -> ("error out"=w105:errorcluster)  [unwired: 7 in, 1 out]
  n101 = call-poly <vilib>:"WPI_MotorControlOpen.vi"("error in (no error)"=w105, "Device Number"=u8 4, "Control Mode"=WPI_CANJaguar_ControlMode."Position") -> ("MotorControlDeviceRef"=w153:T32)  [unwired: 7 in, 1 out]
  n102 = while {
    tunnel: w153 -> [w283]
    tunnel: [w282] -> w152
    tunnel: [w259] -> w107
    tunnel: [w254] -> w99
    i -> [w254]
    stop <- w256 continue-if-true
    w265 = T43 0 items=["Quad Encoder"=0, "Potentiometer"=1, "None"=255] ("Position Reference")
    w279 = T44[] [enum."Position"] items=["Output Percent VBus", "Output Voltage", "Bus Voltage", "Current", "Temperature", "Position", "Speed", "Limit Switches", "Faults", "Fault Counters", "Power Cycle"] ("Status Select")
    # "Assume we start pointed 180 Degrees"
    # "+/- 1 revolutions"
    n103 = call <vilib>:"WPI_CANJaguar_ScheduleStatusUpdates.vi"("Update Period (s)"=0.01, "Status Channel Select"=WPI_CANJaguar_StatusChannelSelect."Periodic Status Channel 3", "Status Select"=w279, "CAN Jaguar Ref"=w283) -> ("error out"=w274:errorcluster, "CAN Jaguar Ref Out"=w275:T32)  [unwired: 6 in]
    n104 = call <vilib>:"WPI_CANJaguar_ConfigEncoderCodesPerRev.vi"("error in (no error)"=w274, "Encoder Codes Per Rev"=u16 128 ("Potentiometer Turns"), "CAN Jaguar Ref"=w275) -> ("error out"=w267:errorcluster, "CAN Jaguar Ref Out"=w266:T32)  [unwired: 7 in]
    n105 = call <vilib>:"WPI_CANJaguar_SetPositionReference.vi"("error in (no error)"=w267, "Position Reference"=w265, "CAN Jaguar Ref"=w266) -> ("error out"=w263:errorcluster, "CAN Jaguar Ref Out"=w264:T32)  [unwired: 7 in]
    n106 = call <vilib>:"WPI_CANJaguar_ConfigLimits.vi"("CAN Jaguar Ref"=w264, "Limit Mode"=WPI_CANJaguar_LimitMode."Soft Position Limits", "Forward Limit Position"=2.75, "Reverse Limit Position"=8.25, "error in (no error)"=w263) -> ("CAN Jaguar Ref Out"=w270:T32, "error out"=w269:errorcluster)  [unwired: 9 in]
    n107 = call <vilib>:"WPI_CANJaguar_SetPID.vi"("CAN Jaguar Ref"=w270, "P"=-1000.0, "I"=-1.0, "D"=0.0, "error in (no error)"=w269) -> ("CAN Jaguar Ref Out"=w277:T32, "error out"=w276:errorcluster)  [unwired: 9 in]
    n108 = call <vilib>:"WPI_MotorControlEnable.vi"("error in (no error)"=w276, "Encoder Initial Position"=5.5, "CAN Jaguar Ref"=w277) -> ("error out"=w259:errorcluster, "CAN Jaguar Ref Out"=w282:T32)  [unwired: 7 in]
    n109 = Unbundle By Name(w259) -> ("status"=w255:bool)
    n110 = Less?(x=w254, y=5) -> (x < y?=w257:bool)
    n111 = And(x=w255, y=w257) -> (x .and. y?=w256:bool)
  }
  n112 = call <vilib>:"WPI_MotorControlRefNum Registry Set.vi"("error in (no error)"=w107, "refnum name"="Turret", "MotorControlDevRef"=w152) -> ("error out"=w104:errorcluster)  [unwired: 7 in, 1 out]
  n113 = call-poly <vilib>:"WPI_MotorControlOpen.vi"("error in (no error)"=w104, "Device Number"=u8 6, "Control Mode"=WPI_CANJaguar_ControlMode."Percent VBus") -> ("error out"=w120:errorcluster, "MotorControlDeviceRef"=w121:T32)  [unwired: 7 in]
  n114 = while {
    tunnel: [w293] -> w122
    tunnel: w121 -> [w292]
    tunnel: w120 -> [w291]
    tunnel: [w285] -> w98
    i -> [w285]
    stop <- w286 continue-if-true
    n115 = call <vilib>:"WPI_CANJaguar_ConfigBrakeCoast.vi"("error in (no error)"=w291, "Brake / Coast Mode"=WPI_CANJaguar_BrakeCoastMode."Coast", "CAN Jaguar Ref"=w292) -> ("error out"=w289:errorcluster, "CAN Jaguar Ref Out"=w293:T32)  [unwired: 7 in]
    n116 = Unbundle By Name(w289) -> ("status"=w284:bool)
    n117 = Less?(x=w285, y=5) -> (x < y?=w287:bool)
    n118 = And(x=w284, y=w287) -> (x .and. y?=w286:bool)
  }
  n119 = call <vilib>:"WPI_MotorControlRefNum Registry Set.vi"("refnum name"="Top Rollers", "MotorControlDevRef"=w122) -> ()  [unwired: 8 in, 2 out]
  n120 = global read "Robot Global Data.vi" "Init Counts"() -> (w103:T45)
  n121 = Bundle By Name(cluster=w103, "Top Shooter"=w101, "Bottom Shooter"=w100, "Turret"=w99, "Stage 2"=w98) -> (w102:T45)
  n122 = global write "Robot Global Data.vi" "Init Counts"(w102) -> ()
